vi "Pokayoka signal.vi"() -> (1 "IL Sensor":T1, 2 "output cluster":T2)   [LabVIEW 2015]
uses:
  Galobal variable_TI.vi
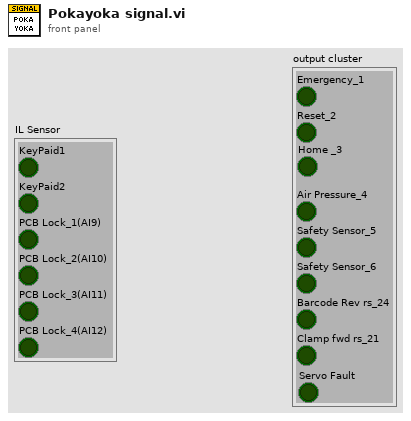
[diagram p1: front panel]
types:
  T1 = cluster{"KeyPaid1":bool, "KeyPaid2":bool, "PCB Lock_1(AI9)":bool, "PCB Lock_2(AI10)":bool, "PCB Lock_3(AI11)":bool, "PCB Lock_4(AI12)":bool}
  T2 = cluster{"Emergency_1":bool, "Reset_2":bool, "Air Pressure_4":bool, "Safety Sensor_5":bool, "Safety Sensor_6":bool, "Barcode Rev rs_24":bool, "Clamp fwd rs_21":bool, "Servo Fault":bool, "Home _3":bool}
  T3 = cluster{"Emergency_1":bool, "Reset_2":bool, "Air Pressure_4":bool, "Safety Sensor_5":bool, "Safety Sensor_6":bool, "Barcode Rev rs_24":bool, "Clamp fwd rs_21":bool, "Servo fault":bool, "Home_3":bool}
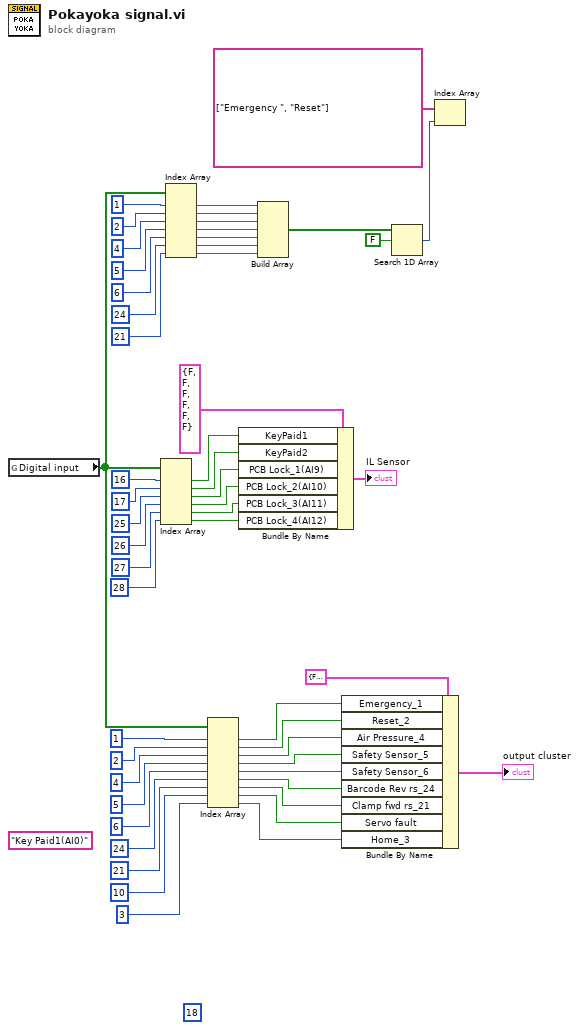
[diagram p0: block diagram]
diagram:
  (unwired) 18 ("index")
  (unwired) "Key Paid1(AI0)"
  n1 = global read "Galobal variable_TI.vi" "Digital input"() -> (w14:bool[])
  n2 = Index Array(array=w14, index #1=16 ("index"), index #2=17 ("index"), index #3=25 ("index"), index #4=26 ("index"), index #5=27 ("index"), index #6=28 ("index")) -> (element #1=w12:bool, element #2=w11:bool, element #3=w10:bool, element #4=w9:bool, element #5=w8:bool, element #6=w7:bool)
  n3 = Index Array(array=w14, index #1=1 ("index"), index #2=2 ("index"), index #3=4 ("index"), index #4=5 ("index"), index #5=6 ("index"), index #6=24 ("index"), index #7=21 ("index")) -> (element #1=w31:bool, element #2=w30:bool, element #3=w29:bool, element #4=w28:bool, element #5=w27:bool, element #6=w26:bool, element #7=w25:bool)
  n4 = Index Array(array=w14, index #1=1 ("index"), index #2=2 ("index"), index #3=4 ("index"), index #4=5 ("index"), index #5=6 ("index"), index #6=24 ("index"), index #7=21 ("index"), index #8=10 ("index"), index #9=3 ("index")) -> (element #1=w53:bool, element #2=w52:bool, element #3=w51:bool, element #4=w50:bool, element #5=w49:bool, element #6=w48:bool, element #7=w47:bool, element #8=w3:bool, element #9=w2:bool)
  n5 = Bundle By Name(cluster=T1 {"KeyPaid1"=FALSE, "KeyPaid2"=FALSE, "PCB Lock_1(AI9)"=FALSE, "PCB Lock_2(AI10)"=FALSE, "PCB Lock_3(AI11)"=FALSE, "PCB Lock_4(AI12)"=FALSE} ("PCB LOCK"), "KeyPaid1"=w12, "KeyPaid2"=w11, "PCB Lock_1(AI9)"=w10, "PCB Lock_2(AI10)"=w9, "PCB Lock_3(AI11)"=w8, "PCB Lock_4(AI12)"=w7) -> (→"IL Sensor":T1)
  n6 = Build Array(w31, w30, w29, w28, w27, w26, w25) -> (w24:bool[])
  n7 = Bundle By Name(cluster=T3 {"Emergency_1"=FALSE, "Reset_2"=FALSE, "Air Pressure_4"=FALSE, "Safety Sensor_5"=FALSE, "Safety Sensor_6"=FALSE, "Barcode Rev rs_24"=FALSE, "Clamp fwd rs_21"=FALSE, "Servo fault"=FALSE, "Home_3"=FALSE} ("Cluster"), "Emergency_1"=w53, "Reset_2"=w52, "Air Pressure_4"=w51, "Safety Sensor_5"=w50, "Safety Sensor_6"=w49, "Barcode Rev rs_24"=w48, "Clamp fwd rs_21"=w47, "Servo fault"=w3, "Home_3"=w2) -> (→"output cluster":T3)
  n8 = Search 1D Array(1D array=w24, element=FALSE) -> (index of element=w22:i32)  [unwired: 1 in]
  n9 = Index Array(array=string[] ["Emergency ", "Reset"], index=w22) -> ()  [unwired: 1 out]
